vi "Arduino-Read.vi"(7 "Arduino function":enum16{"T/RH", "Interlock", "Edgesense"}(ring), 8 "error in (no error)":errorcluster, 9 "Humidity IN":dbl[](array[numeric]), 10 "Temperature IN":dbl[](array[numeric]), 11 "VISA resource name":refnum<visa-resource-name>) -> (0 "error out":errorcluster, 1 "rel. Humidity [%]":dbl, 2 "Temperature [°C]":dbl, 3 "VISA resource name out":refnum<visa-resource-name>, 5 "Edgesense Status":u16(ring)=1 items=["Contact", "No contact"], 6 "Interlock Status":u16(ring) items=["Dark", "Light"])   [LabVIEW 2018]
panel:
  out "Humidity OUT":dbl[](array[numeric])
  out "Temperature OUT":dbl[](array[numeric])
  out "return count":u32
  out "String":string
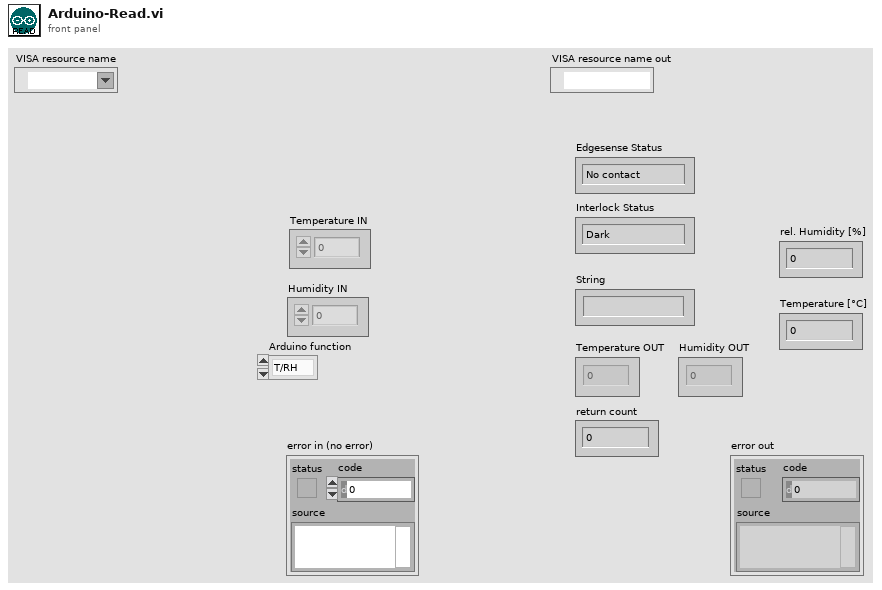
[diagram p1: front panel]
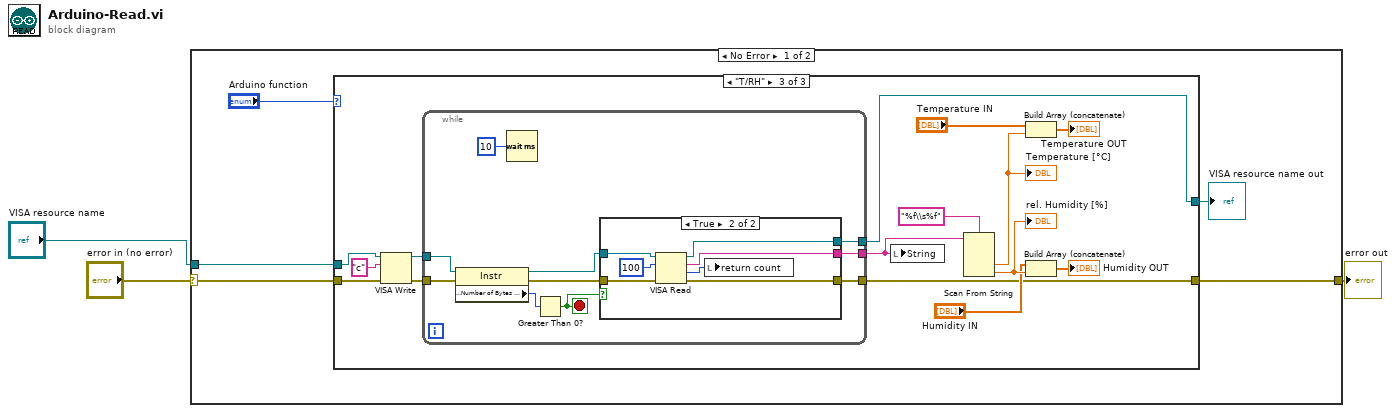
[diagram p0: block diagram]
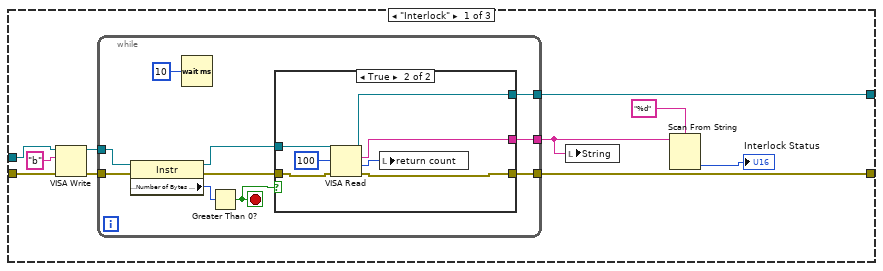
[diagram p2: hidden frame]
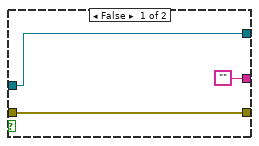
[diagram p3: hidden frame]
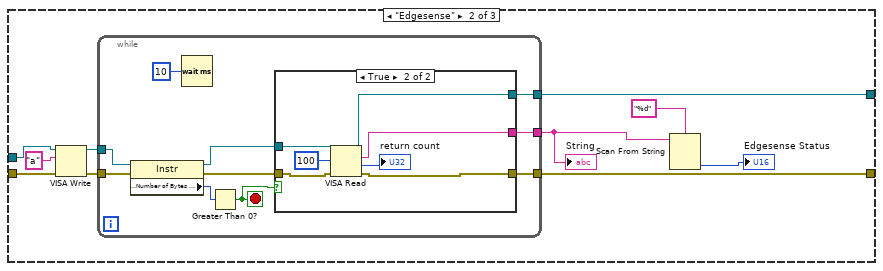
[diagram p4: hidden frame]
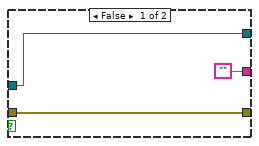
[diagram p5: hidden frame]
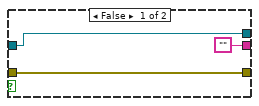
[diagram p6: hidden frame]
diagram:
  n1 = case shown="No Error" "error in (no error)" {
    selector: "error in (no error)" -> [w6 w104]
    tunnel: [w7 w104] -> w2
    tunnel: "VISA resource name" -> [w5 _]
    frame No Error {
      n2 = case shown="\"T/RH\"" "Arduino function" {
        tunnel: w6 -> [w10 w41 w71]
        tunnel: w5 -> [w12 w42 w73]
        tunnel: [w15 w44 w74] -> w4
        tunnel: [w14 w45 w75] -> w7
        frame "Interlock" {
          n3 = VISA Write(VISA resource name=w12, write buffer="b", error in (no error)=w10) -> (VISA resource name out=w11:refnum<visa-resource-name>, error out=w9:errorcluster)  [unwired: 1 out]
          n4 = while {
            tunnel: [w26] -> w15
            tunnel: [w25] -> w16
            tunnel: w9 -> [w19]
            tunnel: w11 -> [w20]
            tunnel: [w24] -> w14
            stop <- w21 stop-if-true
            n5 = property class="Instr"(reference=w20, error in=w19) -> (reference out=w28:refnum<visa-resource-name>, error out=w27:errorcluster, "Serial Settings:Number of Bytes at Serial Port"=w22:u32)
            n6 = Wait (ms)(milliseconds to wait=10) -> ()  [unwired: 1 out]
            n7 = Greater Than 0?(x=w22) -> (x > 0?=w21:bool)
            n8 = case shown="True" w21 {
              tunnel: w28 -> [w29 w38]
              tunnel: w27 -> [w30 w37]
              tunnel: [w29 w36] -> w26
              tunnel: ["" w35] -> w25
              tunnel: [w30 w34] -> w24
              frame False {
              }
              frame True {
                n9 = VISA Read(VISA resource name=w38, byte count=100, error in (no error)=w37) -> (VISA resource name out=w36:refnum<visa-resource-name>, read buffer=w35:string, return count=w33:u32, error out=w34:errorcluster)
                n10 = local write "return count"(w33) -> ()
              }
            }
          }
          n11 = local write "String"(w16) -> ()
          n12 = Scan From String(format string="%d", input string=w16) -> (output 1=→"Interlock Status":u16)  [unwired: 3 in, 3 out]
        }
        frame "Edgesense" {
          n13 = VISA Write(VISA resource name=w42, write buffer="a", error in (no error)=w41) -> (VISA resource name out=w40:refnum<visa-resource-name>, error out=w39:errorcluster)  [unwired: 1 out]
          n14 = while {
            tunnel: [w56] -> w44
            tunnel: [w55] -> w46
            tunnel: w40 -> [w51]
            tunnel: [w54] -> w45
            tunnel: w39 -> [w52]
            stop <- w49 stop-if-true
            n15 = property class="Instr"(reference=w51, error in=w52) -> (reference out=w58:refnum<visa-resource-name>, error out=w57:errorcluster, "Serial Settings:Number of Bytes at Serial Port"=w50:u32)
            n16 = Wait (ms)(milliseconds to wait=10) -> ()  [unwired: 1 out]
            n17 = Greater Than 0?(x=w50) -> (x > 0?=w49:bool)
            n18 = case shown="True" w49 {
              tunnel: w58 -> [w59 w68]
              tunnel: w57 -> [w60 w67]
              tunnel: [w59 w66] -> w56
              tunnel: ["" w65] -> w55
              tunnel: [w60 w64] -> w54
              frame False {
              }
              frame True {
                n19 = VISA Read(VISA resource name=w68, byte count=100, error in (no error)=w67) -> (VISA resource name out=w66:refnum<visa-resource-name>, read buffer=w65:string, return count=→"return count":u32, error out=w64:errorcluster)
              }
            }
          }
          "String" <- w46
          n20 = Scan From String(format string="%d", input string=w46) -> (output 1=→"Edgesense Status":u16)  [unwired: 3 in, 3 out]
        }
        frame "T/RH" {
          n21 = VISA Write(VISA resource name=w73, write buffer="c", error in (no error)=w71) -> (VISA resource name out=w69:refnum<visa-resource-name>, error out=w70:errorcluster)  [unwired: 1 out]
          n22 = while {
            tunnel: [w91] -> w74
            tunnel: [w90] -> w76
            tunnel: w70 -> [w85]
            tunnel: w69 -> [w84]
            tunnel: [w89] -> w75
            stop <- w86 stop-if-true
            n23 = property class="Instr"(reference=w84, error in=w85) -> (reference out=w93:refnum<visa-resource-name>, error out=w92:errorcluster, "Serial Settings:Number of Bytes at Serial Port"=w87:u32)
            n24 = Wait (ms)(milliseconds to wait=10) -> ()  [unwired: 1 out]
            n25 = Greater Than 0?(x=w87) -> (x > 0?=w86:bool)
            n26 = case shown="True" w86 {
              tunnel: w93 -> [w94 w103]
              tunnel: w92 -> [w95 w102]
              tunnel: [w94 w101] -> w91
              tunnel: ["" w100] -> w90
              tunnel: [w95 w99] -> w89
              frame False {
              }
              frame True {
                n27 = VISA Read(VISA resource name=w103, byte count=100, error in (no error)=w102) -> (VISA resource name out=w101:refnum<visa-resource-name>, read buffer=w100:string, return count=w97:u32, error out=w99:errorcluster)
                n28 = local write "return count"(w97) -> ()
              }
            }
          }
          n29 = local write "String"(w76) -> ()
          n30 = Scan From String(format string="%f\\s%f", input string=w76) -> (output 1=w78:dbl, output 2=w83:dbl)  [unwired: 4 in, 3 out]
          "rel. Humidity [%]" <- w83
          "Temperature [°C]" <- w78
          n31 = Build Array (concatenate)("Temperature IN", w78) -> (→"Temperature OUT":dbl[])
          n32 = Build Array (concatenate)("Humidity IN", w83) -> (→"Humidity OUT":dbl[])
        }
      }
      "VISA resource name out" <- w4
    }
    frame Error {
    }
  }
  "error out" <- w2
